vi "Add tab deliminated parameter.vi"(3 "Value":string, 4 "Parameter":string, 5 "Head":string) -> (2 "resulting string":string)   [LabVIEW 2017]
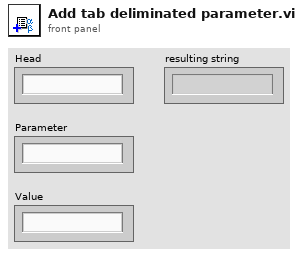
[diagram p1: front panel]
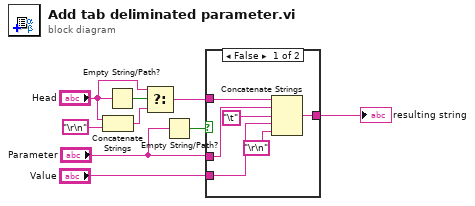
[diagram p0: block diagram]
diagram:
  n1 = Concatenate Strings("Head", "\r\n") -> (w3:string)
  n2 = Empty String/Path?(string/path="Head") -> (empty?=w2:bool)
  n3 = Select(t="Head", s=w2, f=w3) -> (s? t:f=w5:string)
  n4 = Empty String/Path?(string/path="Parameter") -> (empty?=w7:bool)
  n5 = case shown="False" w7 {
    tunnel: "Value" -> [w11 _]
    tunnel: [w14 w16] -> w1
    tunnel: w5 -> [w15 w16]
    tunnel: "Parameter" -> [w13 _]
    frame False {
      n6 = Concatenate Strings(w15, w13, "\t", w11, "\r\n") -> (w14:string)
    }
    frame True {
    }
  }
  "resulting string" <- w1
